vi "ABR3-Plot Traces.vi"(0 "Analysis":T1, 1 "Avg Mode":enum16{"Neural/CM", "ANOW"}(ring), 9 "Normalize individual?":bool, 11 "error in (no error)":errorcluster, 12 "Neural Ref":refnum<vi>, 13 "CM Ref":refnum<vi>) -> (15 "error out":errorcluster)   [LabVIEW 2020]
uses:
  TypeDefs/ABR3-Analysis State.ctl
  Threshold Estimation VIs/ABR3-Threshold Estimation Result.ctl
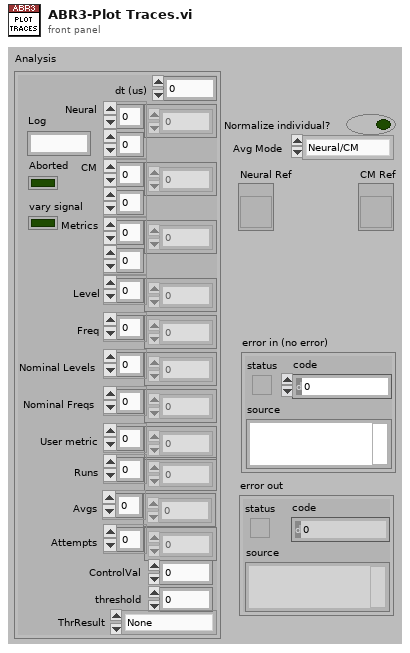
[diagram p1: front panel]
types:
  T1 = typedef "ABR3-Analysis State.ctl" = cluster{"dt (us)":dbl, "Neural":dbl[][], "CM":dbl[][], "Metrics":dbl[][], "Level":dbl[], "Freq":dbl[], "Nominal Levels":dbl[], "Nominal Freqs":dbl[], "User metric":dbl[], "Runs":i32[], "Avgs":i32[], "Attempts":i32[], "Log":string, "Aborted":bool, "ControlVal":dbl, "threshold":dbl, "vary signal":bool, "ThrResult":T2}
  T2 = typedef "ABR3-Threshold Estimation Result.ctl" = enum16{"None", "Power", "Sigmoid", "Power (noisy)", "Suprathreshold", "Invalid"}
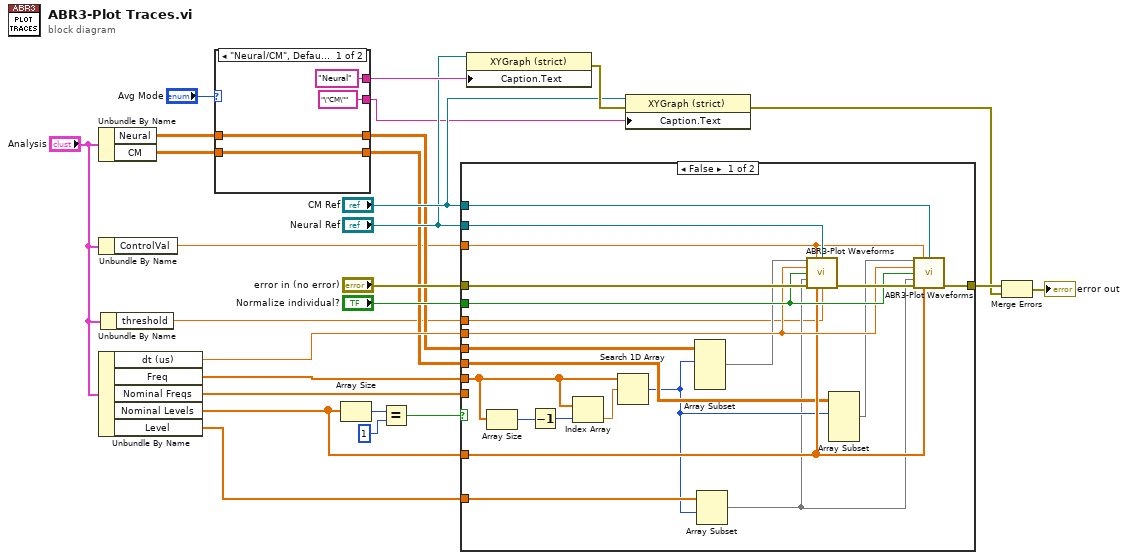
[diagram p0: block diagram]
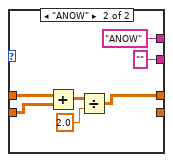
[diagram p2: hidden frame]
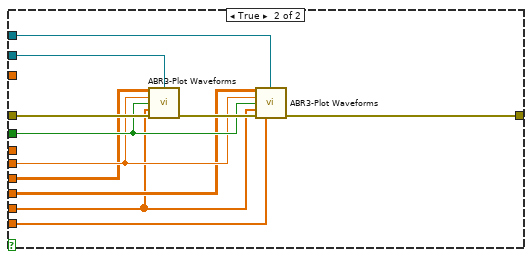
[diagram p3: hidden frame]
diagram:
  n1 = Unbundle By Name("Analysis") -> ("Neural"=w9:dbl[][], "CM"=w8:dbl[][])
  n2 = Unbundle By Name("Analysis") -> ("ControlVal"=w3:dbl)
  n3 = Unbundle By Name("Analysis") -> ("dt (us)"=w23:dbl, "Freq"=w22:dbl[], "Nominal Freqs"=w4:dbl[], "Nominal Levels"=w5:dbl[], "Level"=w19:dbl[])
  n4 = Unbundle By Name("Analysis") -> ("threshold"=w1:dbl)
  n5 = case shown="\"Neural/CM\", Default" "Avg Mode" {
    tunnel: ["Neural" ("Plot.Plot Name") "ANOW" ("Plot.Plot Name")] -> w16
    tunnel: ["\"CM\"" ("Plot.Plot Name") "" ("Plot.Plot Name")] -> w12
    tunnel: w9 -> [w28 w35]
    tunnel: w8 -> [w27 w34]
    tunnel: [w28 w31] -> w7
    tunnel: [w27 _] -> w6
    frame "Neural/CM", Default {
    }
    frame "ANOW" {
      n6 = Add(x=w35, y=w34) -> (x+y=w33:dbl[][])
      n7 = Divide(x=w33, y=2.0) -> (x/y=w31:dbl[][])
    }
  }
  n8 = Array Size(array=w5) -> (size(s)=w21:i32)
  n9 = Equal?(x=w21, y=1 ("x")) -> (x = y?=w26:bool)
  n10 = case shown="False" w26 {
    tunnel: "Neural Ref" -> [w40 w69]
    tunnel: "CM Ref" -> [w41 w68]
    tunnel: "error in (no error)" -> [w56 w66]
    tunnel: "Normalize individual?" -> [w54 w65]
    tunnel: w23 -> [w53 w64]
    tunnel: w7 -> [w50 w63]
    tunnel: w6 -> [w48 w62]
    tunnel: w4 -> [_ w59]
    tunnel: w22 -> [w46 w61]
    tunnel: w5 -> [w52 _]
    tunnel: [w51 w60] -> w20
    tunnel: w19 -> [w44 _]
    tunnel: w3 -> [w39 _]
    tunnel: w1 -> [w38 _]
    frame False {
      n11 = Array Size(array=w46) -> (size(s)=w58:i32)
      n12 = Decrement(x=w58) -> (x-1=w57:i32)
      n13 = Index Array(array=w46, index=w57) -> (element=w45:dbl)
      n14 = Search 1D Array(1D array=w46, element=w45) -> (index of element=w43:i32)  [unwired: 1 in]
      n15 = Array Subset(array=w50, index (row)=w43) -> (w49:dbl[][])  [unwired: 3 in]
      n16 = Array Subset(array=w44, index=w43) -> (w42:dbl[])  [unwired: 1 in]
      n17 = call "ABR3-Plot Waveforms.vi"("Array"=w49, "ControlVal"=w39, "graph ref"=w40, "dt (us)"=w53, "Normalize traces"=w54, "Seqvals"=w42, "error in (no error)"=w56, "InnerVals"=w52, "Threshold"=w38) -> ("error out"=w55:errorcluster)  [unwired: 6 in]
      n18 = Array Subset(array=w48, index (row)=w43) -> (w47:dbl[][])  [unwired: 3 in]
      n19 = call "ABR3-Plot Waveforms.vi"("Array"=w47, "ControlVal"=w39, "graph ref"=w41, "dt (us)"=w53, "Normalize traces"=w54, "Seqvals"=w42, "error in (no error)"=w55, "InnerVals"=w52) -> ("error out"=w51:errorcluster)  [unwired: 7 in]
    }
    frame True {
      n20 = call "ABR3-Plot Waveforms.vi"("Array"=w63, "graph ref"=w69, "dt (us)"=w64, "Normalize traces"=w65, "Seqvals"=w61, "error in (no error)"=w66) -> ("error out"=w67:errorcluster)  [unwired: 9 in]
      n21 = call "ABR3-Plot Waveforms.vi"("Array"=w62, "graph ref"=w68, "dt (us)"=w64, "Normalize traces"=w65, "Seqvals"=w61, "error in (no error)"=w67, "InnerVals"=w59) -> ("error out"=w60:errorcluster)  [unwired: 8 in]
    }
  }
  n22 = property class="XYGraph (strict)"(reference="Neural Ref", "Caption.Text"=w16) -> (error out=w15:errorcluster)  [unwired: 1 in, 1 out]
  n23 = property class="XYGraph (strict)"(reference="CM Ref", error in=w15, "Caption.Text"=w12) -> (error out=w10:errorcluster)  [unwired: 1 out]
  n24 = Merge Errors(w20, w10) -> (→"error out":errorcluster)
